vi "Get Objects.vi"(11 "Component in":refnum<class "Component.lvclass">) -> (2 "objects":refnum<class>[](array[class]), 3 "Component out":refnum<class "Component.lvclass">)   [LabVIEW 2017, in "DSF Core.lvlib" / "Component.lvclass"]
uses:
  Component.lvclass
  Component.lvclass/Component.ctl
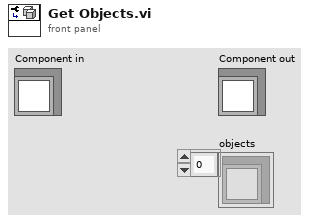
[diagram p1: front panel]
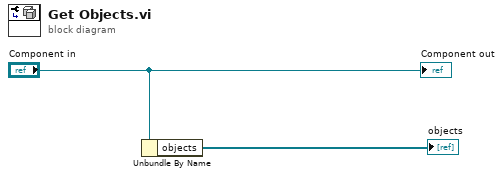
[diagram p0: block diagram]
diagram:
  n1 = Unbundle By Name("Component in") -> ("objects"=→"objects":refnum<class>[])
  "Component out" <- "Component in"
